vi "Compare.vi"() -> ()   [LabVIEW 2020]
uses:
  Utilities/Arguments.ctl
  Screenshots/VIScreenshots.ctl
  Screenshots/ScreenshotInfo.ctl
  Screenshots/Screenshot Type.ctl
  Utilities/FilePaths.ctl
panel:
  out "Output Path In":path
  out "New VI Path In":path
  out "Old VI Path In":path
  out "Error Out":errorcluster
  in  "New VI Path":path
  in  "Old VI Path":path
  in  "Output Path":path
  out "Description":string
  in  "error in":errorcluster
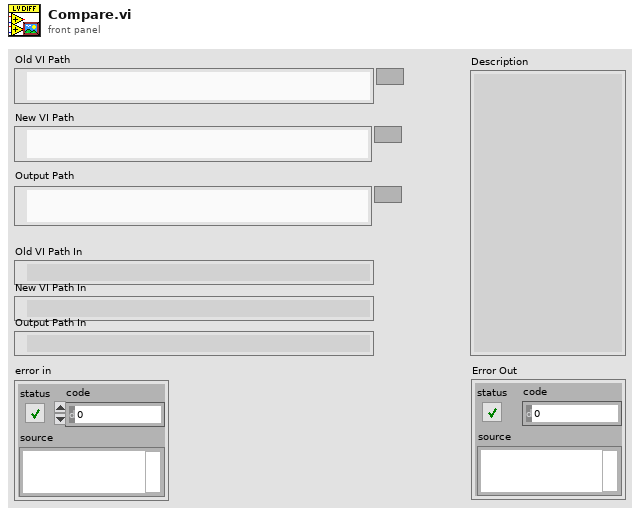
[diagram p1: front panel]
types:
  T1 = typedef "VIScreenshots.ctl" = cluster{"Front Panel Screenshots":T2[], "Block Diagram Screenshots":T2[], "Connector Pane Screenshots":T2[], "VI Hierarchy Screenshots":T2[], "Unknown Screenshots":T2[], "vi reference":refnum<vi>, "File Paths":cluster{"File Path":path, "Container Path":path}, "Name":string}
  T2 = typedef "ScreenshotInfo.ctl" = cluster{"Screenshot Path":path, "Screenshot Type":T3, "VI Paths":T4}
  T3 = typedef "Screenshot Type.ctl" = enum16{"Unknown", "Front Panel", "Connector Pane", "Block Diagram", "VI Hierarchy"}
  T4 = typedef "FilePaths.ctl" = cluster{"File Path":path, "Container Path":path}
  T5 = typedef "Arguments.ctl" = cluster{"VI 1 Path":path, "VI 2 Path":path, "Picture Save Location":path, "Screenshot Title":string}
  T6 = typedef "Output Folders.ctl" = cluster{"combined":path, "vi1shots":path, "vi2shots":path, "Picture Save Location":path}
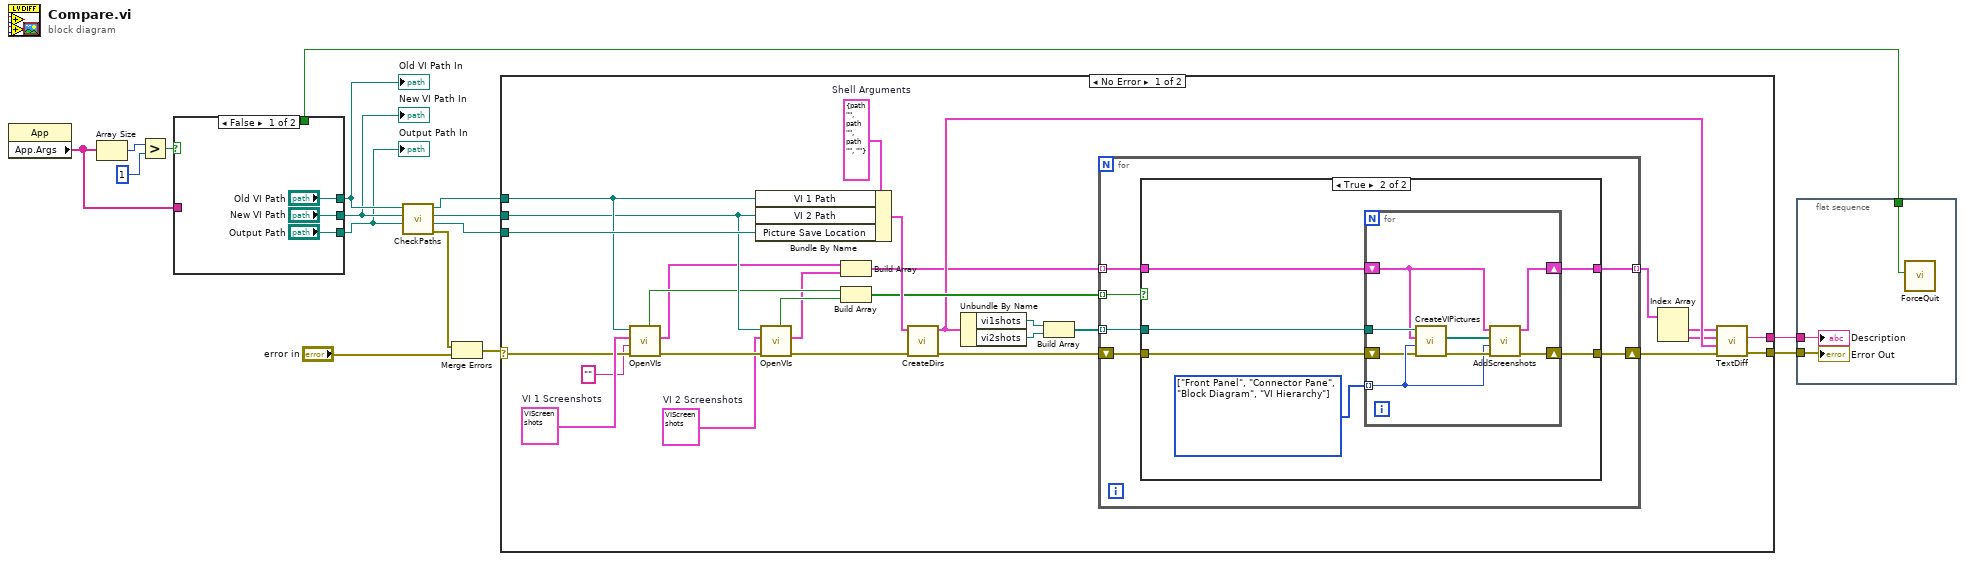
[diagram p0: block diagram]
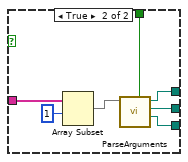
[diagram p2: hidden frame]
diagram:
  n1 = property class="App"() -> ("App.Args"=w5:string[])  [unwired: 2 in, 2 out]
  n2 = Array Size(array=w5) -> (size(s)=w4:i32)
  n3 = Greater?(x=w4, y=1) -> (0:w3:bool)
  n4 = case shown="False" w3 {
    tunnel: ["Old VI Path" w26] -> w11
    tunnel: ["New VI Path" w25] -> w10
    tunnel: ["Output Path" w24] -> w9
    tunnel: w5 -> [_ w23]
    tunnel: [_ w20] -> w1
    frame False {
    }
    frame True {
      n5 = Array Subset(array=w23, index=1) -> (w22:string[])  [unwired: 1 in]
      n6 = call "ParseArguments.vi"("Arguments"=w22) -> ("Output Path"=w24:path, "New VI Path"=w25:path, "Old VI Path"=w26:path, "Boolean"=w20:bool)  [unwired: 7 in]
    }
  }
  "Old VI Path In" <- w11
  "New VI Path In" <- w10
  "Output Path In" <- w9
  n7 = call "CheckPaths.vi"("Output Path"=w9, "New VI Path"=w10, "Old VI Path"=w11) -> ("error out"=w12:errorcluster, "Output Path Out"=w6:path, "New VI Path Out"=w7:path, "Old VI Path Out"=w8:path)  [unwired: 5 in]
  n8 = Merge Errors(w12, "error in") -> (w14:errorcluster)
  n9 = case shown="No Error" w14 {
    selector: w14 -> [w44 w77]
    tunnel: w6 -> [w53 _]
    tunnel: [w50 _] -> w16
    tunnel: [w49 w77] -> w13
    tunnel: w8 -> [w48 _]
    tunnel: w7 -> [w46 _]
    frame No Error {
      w42 = T1 {"Front Panel Screenshots"=[], "Block Diagram Screenshots"=[], "Connector Pane Screenshots"=[], "VI Hierarchy Screenshots"=[], "Unknown Screenshots"=[], "vi reference"=refnum, "File Paths"={"File Path"=path "", "Container Path"=path ""}, "Name"=""}  # VI 2 Screenshots
      w51 = T1 {"Front Panel Screenshots"=[], "Block Diagram Screenshots"=[], "Connector Pane Screenshots"=[], "VI Hierarchy Screenshots"=[], "Unknown Screenshots"=[], "vi reference"=refnum, "File Paths"={"File Path"=path "", "Container Path"=path ""}, "Name"=""}  # VI 1 Screenshots
      w54 = T5 {"VI 1 Path"=path "", "VI 2 Path"=path "", "Picture Save Location"=path "", "Screenshot Title"=""}  # Shell Arguments
      n10 = call "OpenVIs.vi"("error in (no error)"=w44, "Title Prefix In"="", "VI Screenshots"=w51, "VI Path"=w48) -> ("error out"=w45:errorcluster, "VI Screenshots out"=w33:T1, "VI exists?"=w41:bool)  [unwired: 5 in]
      n11 = Bundle By Name(cluster=w54, "VI 1 Path"=w48, "VI 2 Path"=w46, "Picture Save Location"=w53) -> (w52:T5)
      n12 = call "OpenVIs.vi"("error in (no error)"=w45, "VI Screenshots"=w42, "VI Path"=w46) -> ("error out"=w47:errorcluster, "VI Screenshots out"=w34:T1, "VI exists?"=w40:bool)  [unwired: 6 in]
      n13 = Build Array(w33, w34) -> (w32:T1[])
      n14 = Build Array(w41, w40) -> (w39:bool[])
      n15 = call "CreateDirs.vi"("error in (no error)"=w47, "Shell Arguments"=w52) -> ("error out"=w31:errorcluster, "Output Folders"=w38:T6)  [unwired: 8 in]
      n16 = Unbundle By Name(w38) -> ("vi1shots"=w37:path, "vi2shots"=w36:path)
      n17 = Build Array(w37, w36) -> (w35:path[])
      n18 = for {
        tunnel: w39 -> [w60] mode=indexing
        tunnel: w35 -> [w59] mode=indexing
        tunnel: w32 -> [w58] mode=indexing
        shift-right: [w56] -> w27
        shift-left: w31 -> [w57]
        tunnel: [w55] -> w30 mode=indexing
        n19 = case shown="True" w60 {
          tunnel: w59 -> [_ w67]
          tunnel: w58 -> [w62 w66]
          tunnel: w57 -> [w61 w65]
          tunnel: [w61 w64] -> w56
          tunnel: [w62 w63] -> w55
          frame False {
          }
          frame True {
            w68 = T3[] [enum."Front Panel", enum."Connector Pane", enum."Block Diagram", enum."VI Hierarchy"] items=["Unknown", "Front Panel", "Connector Pane", "Block Diagram", "VI Hierarchy"]
            n20 = for {
              tunnel: w68 -> [w74] mode=indexing
              tunnel: w67 -> [w73]
              shift-right: [w71] -> w63
              shift-left: w66 -> [w72]
              shift-right: [w69] -> w64
              shift-left: w65 -> [w70]
              n21 = call "CreateVIPictures.vi"("error in (no error)"=w70, "Capture Target"=w74, "VI Screenshots"=w72, "Picture Save Location"=w73) -> ("error out"=w75:errorcluster, "Screenshot Files"=w76:path[])  [unwired: 6 in]
              n22 = call "AddScreenshots.vi"("error in (no error)"=w75, "Screenshot Type"=w74, "Screenshot Paths"=w76, "VI Screenshots In"=w72) -> ("error out"=w69:errorcluster, "VI Screenshots Out"=w71:T1)  [unwired: 6 in]
            }
          }
        }
      }
      n23 = Index Array(array=w30) -> (element #1=w29:T1, element #2=w28:T1)  [unwired: 2 in]
      n24 = call "TextDiff.vi"("error in (no error)"=w27, "Output Folders"=w38, "VI 2 Screenshots in"=w28, "VI 1 Screenshots in"=w29) -> ("error out"=w49:errorcluster, "Description"=w50:string)  [unwired: 6 in]
    }
    frame Error {
    }
  }
  n25 = flat-sequence {
    tunnel: w16 -> [w80]
    tunnel: w13 -> [w79]
    tunnel: w1 -> [w78]
    frame #0 {
      n26 = call "ForceQuit.vi"("Quit (T)"=w78) -> ()  [unwired: 9 in, 2 out]
      "Description" <- w80
      "Error Out" <- w79
    }
  }
